vi "sensoresflag.vi"(0 "NXT IN":T1) -> (1 "NXT OUT":T1, 2 "FinalizarPrograma?":bool)   [LabVIEW 2015, in "ExemploFinal.lvrbt"]
uses:
  ExemploFinal.lvrbt
  <vilib>/NXT/Subs/LVHSConnector.ctl
  <vilib>/NXT/LegoClasses/BrickReference/BrickReference.lvclass
  <vilib>/NXT/Block Support/NXT_ButtonSelector.ctl
  <vilib>/NXT/Block Support/NXT_InputPort.ctl
  <vilib>/NXT/Dual Mode Library/Sensors/Touch_Pressed.vi
  <vilib>/NXT/Dual Mode Library/Sensors/readNXTButton.vi
  <vilib>/NXT/Dual Mode Library/Sensors/Sonar_cm.vi
  <vilib>/NXT/Dual Mode Library/Sensors/Color_None.vi
  <vilib>/NXT/Dual Mode Library/Sensors/Sound_dBA.vi
panel:
  # "Este VI apenas verifica o estado dos sensores e grava seus valores nem flags para futuras utilizações.\nMensagens são gravadas em flags também para apresentações no visor do NXT 2.0."
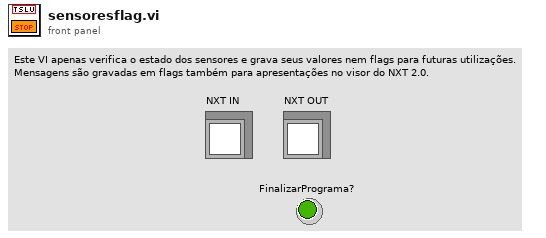
[diagram p1: front panel]
types:
  T1 = typedef "LVHSConnector.ctl" = refnum<class "BrickReference.lvclass">
  T2 = cluster{"TouchIN":bool, "SomIN":i16, "LuzIN":i16, "UltrasomIN":i16, "BotãoIN":bool}
  T3 = typedef "NXT_InputPort.ctl" = u32
  T4 = typedef "NXT_ButtonSelector.ctl" = u16
  T5 = cluster{"TouchOUT":bool, "SomOUT":i32, "LuzOUT":i32, "UltrasomOUT":i32, "BotãoOUT":bool}
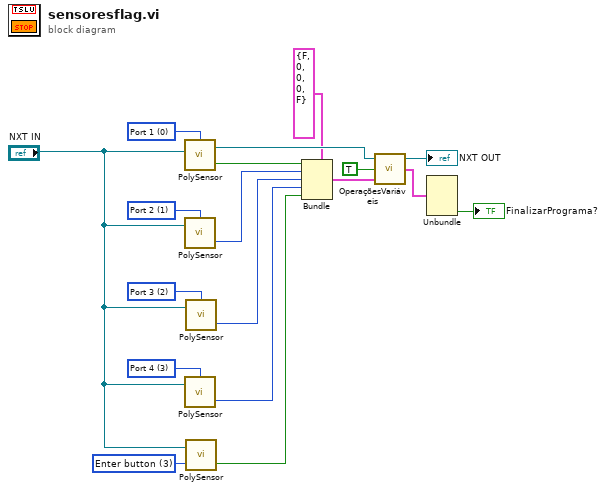
[diagram p0: block diagram]
diagram:
  w14 = T3 0 items=["Port 1", "Port 2", "Port 3", "Port 4"] ("Port (Port 1)")
  w15 = T3 1 items=["Port 1", "Port 2", "Port 3", "Port 4"] ("Port (Port 2)")
  w16 = T3 2 items=["Port 1", "Port 2", "Port 3", "Port 4"] ("Port (Port 3)")
  w17 = T3 3 items=["Port 1", "Port 2", "Port 3", "Port 4"] ("Port (Port 4)")
  w18 = T4 3 items=["Enter button"=3, "Left button"=2, "Right button"=1, "Up Button"=4, "Down Button"=5] ("Button (Enter button)")
  n1 = call-poly <vilib>:"PolySensor.vi"("NXT/EV3"="NXT IN", "Port (Port 1)"=w14) -> ("Yes / No"=w7:bool, "NXT/EV3"=w6:T1)  [unwired: 1 in]
  n2 = call-poly <vilib>:"PolySensor.vi"("NXT/EV3"="NXT IN", "Port (Port 2)"=w15) -> ("sound (dBA)"=w8:i16)  [unwired: 1 in, 1 out]
  n3 = call-poly <vilib>:"PolySensor.vi"("NXT/EV3"="NXT IN", "Port (Port 4)"=w17) -> ("Distance (cm)"=w10:i16)  [unwired: 1 in, 1 out]
  n4 = call-poly <vilib>:"PolySensor.vi"("NXT/EV3"="NXT IN", "Port (Port 3)"=w16) -> ("Scaled Value"=w9:i16)  [unwired: 1 in, 1 out]
  n5 = call-poly <vilib>:"PolySensor.vi"("Button (Enter button)"=w18, "NXT/EV3"="NXT IN") -> ("Yes/No"=w11:bool)  [unwired: 1 in, 1 out]
  n6 = Bundle(cluster=T2 {"TouchIN"=FALSE, "SomIN"=0, "LuzIN"=0, "UltrasomIN"=0, "BotãoIN"=FALSE} ("Entradas"), "TouchIN"=w7, "SomIN"=w8, "LuzIN"=w9, "UltrasomIN"=w10, "BotãoIN"=w11) -> (w2:T2)
  n7 = call "OperaçõesVariáveis.vi"("Entradas"=w2, "Escrever?"=TRUE, "NXT IN"=w6) -> ("Saídas"=w4:T5, "NXT OUT"=→"NXT OUT":T1)  [unwired: 1 out]
  n8 = Unbundle(w4) -> ("BotãoOUT"=→"FinalizarPrograma?":bool)  [unwired: 4 out]
